vi "AddGroup Value Change.vi"(11 "References":T1) -> (0 "error out":errorcluster)   [LabVIEW 2015, in "TDMS datalogger editor node.lvclass"]
uses:
  TDMS datalogger editor node.lvclass
  <vilib>/NI/DCAF/Tag Editor Core/Table API/Table Manager/object ref.ctl
  <vilib>/NI/DCAF/Tag Editor Core/Configuration Editor/Classes/Engine Parent/Engine Parent Editor Node.lvclass
  <vilib>/NI/DCAF/Tag Editor Core/Configuration Editor/Classes/Module editor node/module editor node.lvclass
  TDMS datalogger editor node.lvclass/TDMS datalogger editor node.ctl
  <vilib>/NI/DCAF/Tag Editor Core/Table API/Table Manager/Table Manager.lvclass
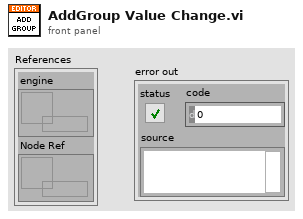
[diagram p1: front panel]
types:
  T1 = typedef "Table Manager.lvlib/Table Manager.lvclass/object ref.ctl" = cluster{"engine":refnum<data-value>, "Node Ref":refnum<data-value>}
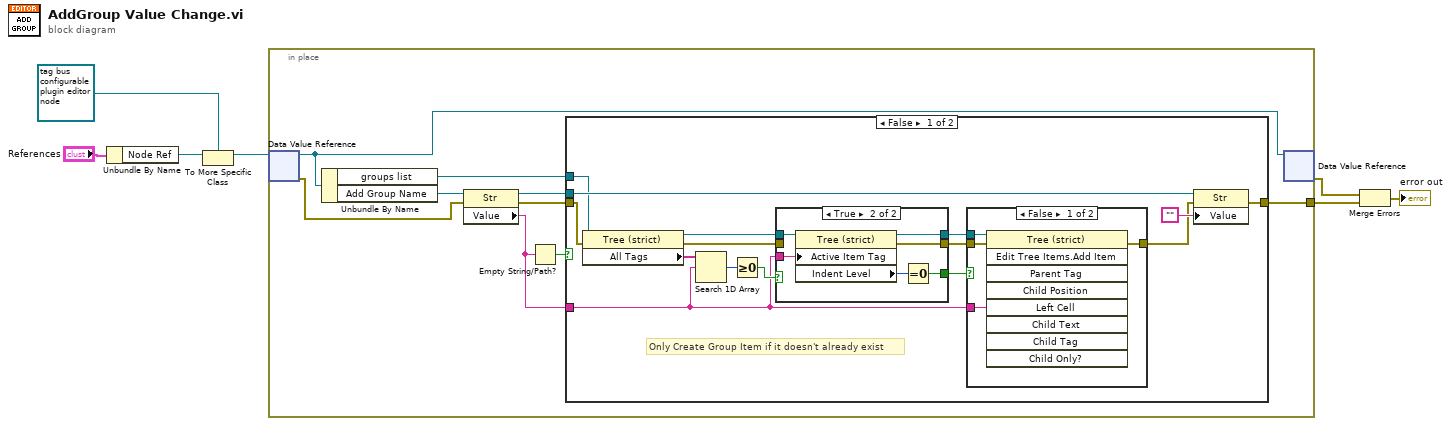
[diagram p0: block diagram]
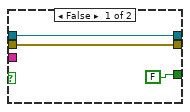
[diagram p3: hidden frame]
diagram:
  n1 = Unbundle By Name("References") -> ("Node Ref"=w5:refnum<data-value>)
  n2 = To More Specific Class(target class=refnum<data-value> refnum ("data value reference"), reference=w5) -> (specific class reference=w3:refnum<data-value>)  [unwired: 1 in, 1 out]
  n3 = in-place {
    in-place-border: [w11] -> w2
    n4 = in-place-dvr #1(w3) -> (w12:refnum<class "TDMS datalogger editor node.lvclass">, w15:errorcluster)
    n5 = Unbundle By Name(w12) -> ("groups list"=w14:refnum<vi>, "Add Group Name"=w16:refnum<vi>)
    n6 = property class="Str"(reference=w16, error in=w15) -> (reference out=w10:refnum<vi>, error out=w13:errorcluster, "Value"=w8:string)
    n7 = Empty String/Path?(string/path=w8) -> (empty?=w9:bool)
    n8 = case shown="False" w9 {
      tunnel: w8 -> [w17 _]
      tunnel: w14 -> [w18 _]
      tunnel: w13 -> [w19 w46]
      tunnel: [w31 w46] -> w11
      tunnel: w10 -> [w29 _]
      frame False {
        # "Only Create Group Item if it doesn't already exist"
        n9 = property class="Tree (strict)"(reference=w18, error in=w19) -> (reference out=w25:refnum<vi>, error out=w28:errorcluster, "All Tags"=w21:string[])
        n10 = Search 1D Array(1D array=w21, element=w17) -> (index of element=w22:i32)  [unwired: 1 in]
        n11 = Greater Or Equal To 0?(x=w22) -> (x >= 0?=w23:bool)
        n12 = case shown="True" w23 {
          tunnel: w17 -> [_ w45]
          tunnel: [FALSE w43] -> w24
          tunnel: w25 -> [w39 w42]
          tunnel: [w39 w41] -> w26
          tunnel: [w37 w40] -> w27
          tunnel: w28 -> [w37 _]
          frame False {
          }
          frame True {
            n13 = property class="Tree (strict)"(reference=w42, "Active Item Tag"=w45) -> (reference out=w41:refnum<vi>, error out=w40:errorcluster, "Indent Level"=w44:i32)  [unwired: 1 in]
            n14 = Equal To 0?(x=w44) -> (x = 0?=w43:bool)
          }
        }
        n15 = case shown="False" w24 {
          tunnel: [w35 w36] -> w20
          tunnel: w17 -> [w34 _]
          tunnel: w26 -> [w33 _]
          tunnel: w27 -> [w32 w36]
          frame False {
            n16 = invoke class="Tree (strict)" method="Edit Tree Items.Add Item"(reference=w33, error in=w32, "Left Cell"=w34) -> (error out=w35:errorcluster)  [unwired: 6 in, 8 out]
          }
          frame True {
          }
        }
        n17 = property class="Str"(reference=w29, error in=w20, "Value"="") -> (error out=w31:errorcluster)  [unwired: 1 out]
      }
      frame True {
        # "Don't add Groups for empty Group Name"
      }
    }
    n18 = in-place-dvr #1(w12) -> (w7:errorcluster)  [unwired: 1 out]
  }
  n19 = Merge Errors(w7, w2) -> (→"error out":errorcluster)
